vi "Data.Result Numeric Look Up Limits.vi"(4 "Limits":variant, 7 "Measurement":T1 {"Status" items=["LOG", "PASS", "FAIL", "ERROR"]}) -> (2 "Measurement Out":T1 {"Status" items=["LOG", "PASS", "FAIL", "ERROR"]})   [LabVIEW 2024, in "EQMF.lvlib" / "Data.lvlib"]
uses:
  Data.lvlib
  TypeDefs/Data.Result Numeric.ctl
  TypeDefs/Data.Result Numeric Limit Type.ctl
  TypeDefs/Data.Result Item Status.ctl
  TypeDefs/Data.Result Limit Definition.ctl
  TypeDefs/Data.Result Numeric Limit Type with Limits.ctl
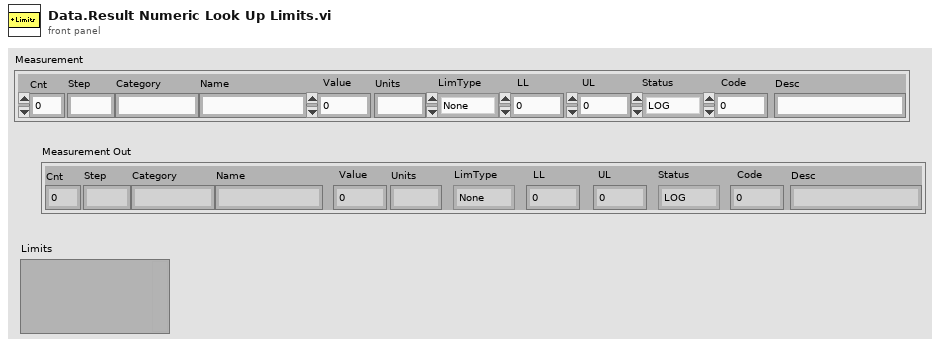
[diagram p1: front panel]
types:
  T1 = typedef "EQMF.lvlib/Data.lvlib/Data.Result Numeric.ctl" = cluster{"Cnt":i32, "Step":string, "Category":string, "Name":string, "Value":dbl, "Units":string, "LimType":T2, "LL":dbl, "UL":dbl, "Status":T3, "Code":i32, "Desc":string}
  T2 = typedef "EQMF.lvlib/Data.lvlib/Data.Result Numeric Limit Type.ctl" = enum16{"None", "EQ", "NE", "GT", "LT", "GE", "LE", "GTLT", "GELE", "GELT", "GTLE", "LTGT", "LEGE", "LEGT", "LTGE"}
  T3 = typedef "EQMF.lvlib/Data.lvlib/Data.Result Item Status.ctl" = i32
  T4 = typedef "EQMF.lvlib/Data.lvlib/Data.Result Limit Definition.ctl" = cluster{"Name":string, "LimType":T2, "LL":dbl, "UL":dbl, "Units":string, "FailCode":i32, "FailDesc":string}
  T5 = typedef "EQMF.lvlib/Data.lvlib/Data.Result Numeric Limit Type with Limits.ctl" = cluster{"LimType":T2, "LL":dbl, "UL":dbl}
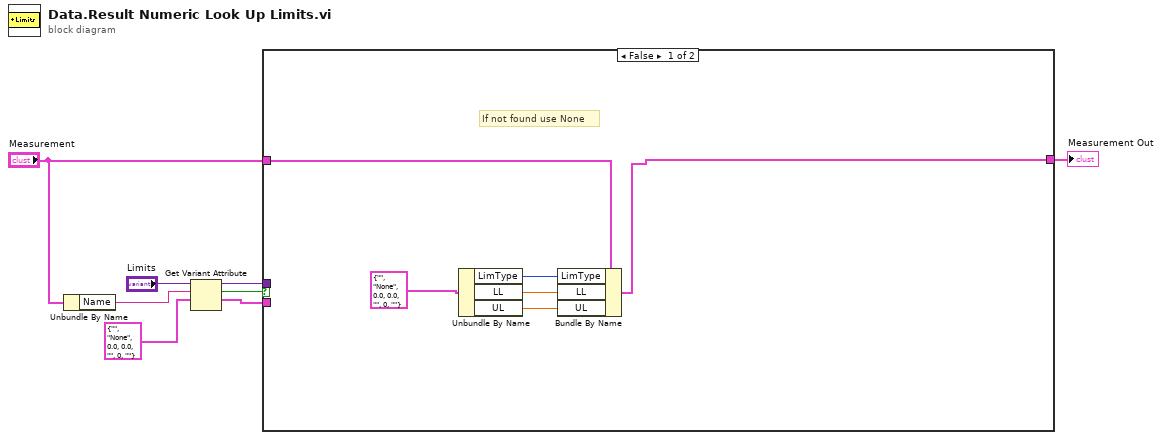
[diagram p0: block diagram]
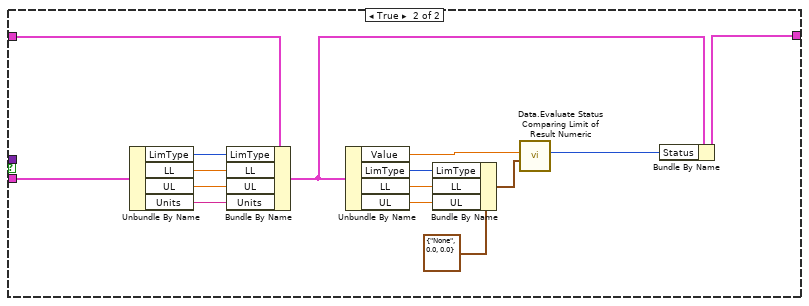
[diagram p2: hidden frame]
diagram:
  n1 = Unbundle By Name("Measurement") -> ("Name"=w7:string)
  n2 = Get Variant Attribute(Variant="Limits", name=w7, default value (empty Variant)=T4 {"Name"="", "LimType"=enum."None", "LL"=0.0, "UL"=0.0, "Units"="", "FailCode"=0, "FailDesc"=""} ("Data.lvlib:Data.Result Limit Definition")) -> (duplicate Variant=w5:variant, found=w6:bool, value=w4:T4)  [unwired: 1 in, 1 out]
  n3 = case shown="False" w6 {
    tunnel: w5 -> [_ _]
    tunnel: w4 -> [_ w25]
    tunnel: "Measurement" -> [w10 w22]
    tunnel: [w9 w21] -> w2
    frame False {
      # "If not found use None"
      n4 = Unbundle By Name(T4 {"Name"="", "LimType"=enum."None", "LL"=0.0, "UL"=0.0, "Units"="", "FailCode"=0, "FailDesc"=""} ("Data.lvlib:Data.Result Limit Definition")) -> ("LimType"=w12:T2, "LL"=w13:dbl, "UL"=w14:dbl)
      n5 = Bundle By Name(cluster=w10, "LimType"=w12, "LL"=w13, "UL"=w14) -> (w9:T1)
    }
    frame True {
      n6 = Unbundle By Name(w25) -> ("LimType"=w26:T2, "LL"=w28:dbl, "UL"=w29:dbl, "Units"=w27:string)
      n7 = Bundle By Name(cluster=w22, "LimType"=w26, "LL"=w28, "UL"=w29, "Units"=w27) -> (w20:T1)
      n8 = Unbundle By Name(w20) -> ("Value"=w23:dbl, "LimType"=w17:T2, "LL"=w18:dbl, "UL"=w16:dbl)
      n9 = Bundle By Name(cluster=T5 {"LimType"=enum."None", "LL"=0.0, "UL"=0.0} ("Limit Def"), "LimType"=w17, "LL"=w18, "UL"=w16) -> (w15:T5)
      n10 = call "Data.Evaluate Status Comparing Limit of Result Numeric.vi"("Limit Def"=w15, "Value"=w23) -> ("Status"=w24:T3)  [unwired: 8 in, 1 out]
      n11 = Bundle By Name(cluster=w20, "Status"=w24) -> (w21:T1)
    }
  }
  "Measurement Out" <- w2
